vi "StandAloneApp.vi"() -> ()   [LabVIEW 2016]
uses:
  VIs/ColorText/Code.xctl
panel:
  in  "Tab Control":enum32{"IntroPage", "Choose"}(tab)
  in  "MoveOn":bool
  in  "Run":bool
  out "Code":string(xcontrol)
  in  "Backpack?":bool
  in  "Spike?":bool
  in  "Templates":i32(listbox)
  in  "Spike Name":string="Select"
  in  "Backpack":string="Select"
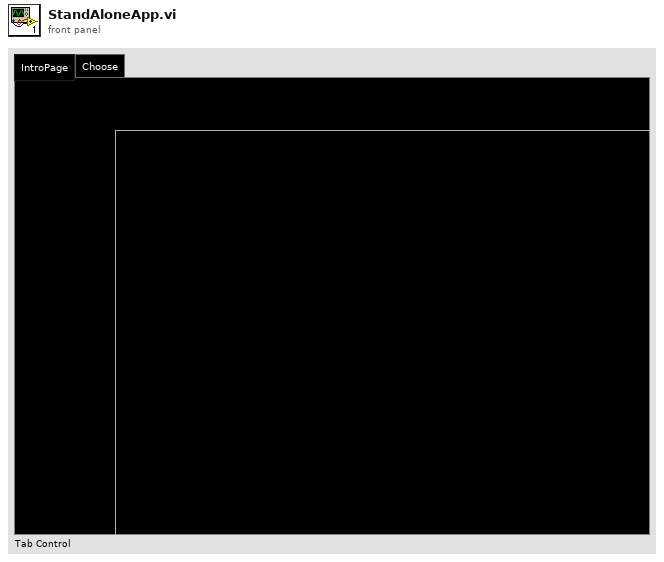
[diagram p1: front panel]
types:
  T1 = enum8{"Enabled", "Disabled", "Disabled and Grayed Out"}
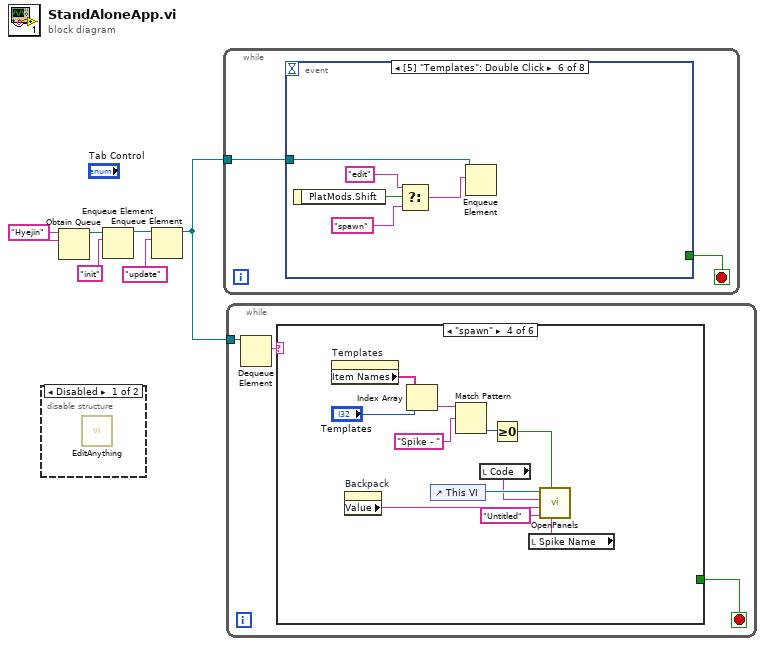
[diagram p0: block diagram]
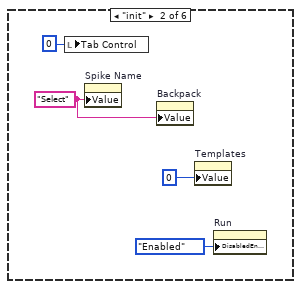
[diagram p4: hidden frame]
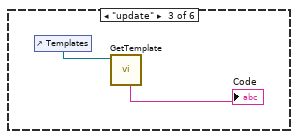
[diagram p5: hidden frame]
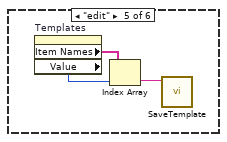
[diagram p6: hidden frame]
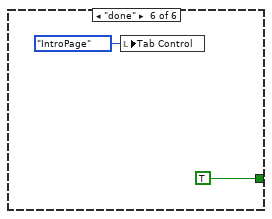
[diagram p7: hidden frame]
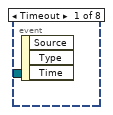
[diagram p8: hidden frame]
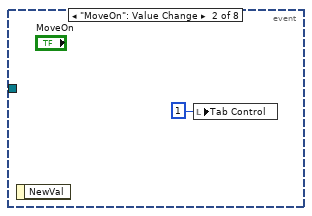
[diagram p9: hidden frame]
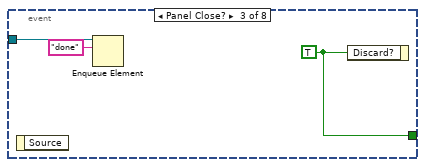
[diagram p10: hidden frame]
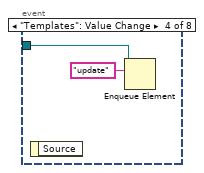
[diagram p11: hidden frame]
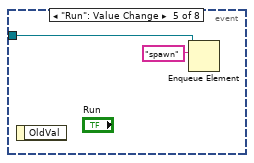
[diagram p12: hidden frame]
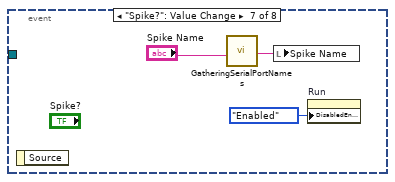
[diagram p13: hidden frame]
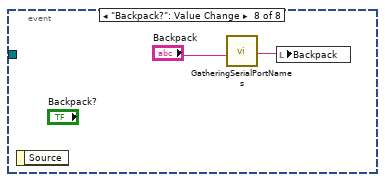
[diagram p14: hidden frame]
diagram:
  w4 = "Hyejin" ("name (unnamed)")
  n1 = disable-structure shown="Disabled" {
    frame Disabled {
      n2 = call "EditAnything.vi"() -> ()  [unwired: 12 in]
    }
    frame Enabled {
    }
  }
  n3 = Obtain Queue(name (unnamed)=w4, element data type=w4) -> (queue out=w6:refnum<queue>)  [unwired: 3 in, 2 out]
  n4 = Enqueue Element(queue=w6, element="init") -> (queue out=w3:refnum<queue>)  [unwired: 2 in, 2 out]
  n5 = Enqueue Element(queue=w3, element="update") -> (queue out=w2:refnum<queue>)  [unwired: 2 in, 2 out]
  n6 = while {
    tunnel: w2 -> [w7]
    stop <- w8 stop-if-true
    n7 = event shown="[5] \"Templates\": Double Click" {
      selector: _ -> [_ _ _ _ _ _ _ _]
      dyn-events: _ -> [_ _ _ _ _ _ _ _]
      timeout: _ -> [_ _ _ _ _ _ _ _]
      tunnel: [_ _ w12 _ _ _ _ _] -> w8
      tunnel: w7 -> [_ _ w10 w13 w15 w21 _ _]
      event Timeout {
        n8 = event-data() -> ()  [unwired: 1 in, 3 out]
      }
      event "MoveOn": Value Change {
        n9 = event-data() -> ()  [unwired: 1 in, 1 out]
        n10 = local write "Tab Control"(1) -> ()
      }
      event Panel Close? {
        w12 = TRUE ("Discard?")
        n11 = event-data() -> ()  [unwired: 1 in, 1 out]
        n12 = Enqueue Element(queue=w10, element="done") -> ()  [unwired: 2 in, 3 out]
        n13 = event-data("Discard?"=w12) -> ()  [unwired: 1 in, 1 out]
      }
      event "Templates": Value Change {
        n14 = event-data() -> ()  [unwired: 1 in, 1 out]
        n15 = Enqueue Element(queue=w13, element="update") -> ()  [unwired: 2 in, 3 out]
      }
      event "Run": Value Change {
        n16 = event-data() -> ()  [unwired: 1 in, 1 out]
        n17 = Enqueue Element(queue=w15, element="spawn") -> ()  [unwired: 2 in, 3 out]
      }
      event "Templates": Double Click {
        n18 = event-data() -> ("PlatMods.Shift"=w20:bool)  [unwired: 1 in]
        n19 = Select(t="edit" ("element"), s=w20, f="spawn" ("element")) -> (s? t:f=w17:string)
        n20 = Enqueue Element(queue=w21, element=w17) -> ()  [unwired: 2 in, 3 out]
      }
      event "Spike?": Value Change {
        n21 = event-data() -> ()  [unwired: 1 in, 1 out]
        n22 = call "GatheringSerialPortNames.vi"("old Name"="Spike Name") -> ("name"=w23:string)  [unwired: 10 in]
        n23 = local write "Spike Name"(w23) -> ()
        n24 = property on="Run" class="Bool"("DisabledEnum"=T1."Enabled" ("Disabled")) -> ()  [unwired: 2 in, 2 out]
      }
      event "Backpack?": Value Change {
        n25 = event-data() -> ()  [unwired: 1 in, 1 out]
        n26 = call "GatheringSerialPortNames.vi"("old Name"="Backpack") -> ("name"=w25:string)  [unwired: 10 in]
        n27 = local write "Backpack"(w25) -> ()
      }
    }
  }
  n28 = while {
    tunnel: w2 -> [w28]
    stop <- w27 stop-if-true
    n29 = Dequeue Element(queue=w28) -> (element=w29:string)  [unwired: 2 in, 3 out]
    n30 = case shown="\"spawn\"" w29 {
      tunnel: [_ _ _ _ _ TRUE ("Discard?")] -> w27
      frame Default {
      }
      frame "init" {
        w32 = "Select" ("Value")
        n31 = local write "Tab Control"(0) -> ()
        n32 = property on="Spike Name" class="Str"("Value"=w32) -> ()  [unwired: 2 in, 2 out]
        n33 = property on="Backpack" class="Str"("Value"=w32) -> ()  [unwired: 2 in, 2 out]
        n34 = property on="Templates" class="LstBox (strict)"("Value"=0 ("Value (Signaling)")) -> ()  [unwired: 2 in, 2 out]
        n35 = property on="Run" class="Bool"("DisabledEnum"=T1."Enabled" ("Disabled")) -> ()  [unwired: 2 in, 2 out]
      }
      frame "update" {
        n36 = control-ref of="Templates"() -> (w35:refnum<vi>)
        n37 = call "GetTemplate.vi"("ListBox in"=w35) -> ("Python"=→"Code":string)  [unwired: 10 in]
      }
      frame "spawn" {
        n38 = property on="Templates" class="LstBox (strict)"() -> ("Item Names"=w41:string[])  [unwired: 2 in, 2 out]
        n39 = property on="Backpack" class="Str"() -> ("Value"=w43:string)  [unwired: 2 in, 2 out]
        n40 = Index Array(array=w41, index="Templates") -> (element=w37:string)
        n41 = control-ref of="This VI"() -> (w46:refnum<vi>)
        n42 = Match Pattern(string=w37, regular expression="Spike - ") -> (offset past match=w39:i32)  [unwired: 1 in, 3 out]
        n43 = local read "Code"() -> (w45:string)
        n44 = Greater Or Equal To 0?(x=w39) -> (x >= 0?=w36:bool)
        n45 = local read "Spike Name"() -> (w44:string)
        n46 = call "OpenPanels.vi"("Spike"=w44, "Single?"=w36, "File Name"="Untitled", "Backpack"=w43, "Code"=w45, "VI in"=w46) -> ()  [unwired: 6 in]
      }
      frame "edit" {
        n47 = property on="Templates" class="LstBox (strict)"() -> ("Item Names"=w49:string[], "Value"=w48:i32)  [unwired: 2 in, 2 out]
        n48 = Index Array(array=w49, index=w48) -> (element=w47:string)
        n49 = call "SaveTemplate.vi"("Template Name"=w47) -> ()  [unwired: 11 in]
      }
      frame "done" {
        n50 = local write "Tab Control"(enum32{"IntroPage", "Choose"}."IntroPage" ("Tab Control")) -> ()
      }
    }
  }
